vi "Get SMO Name.vi"(8 "error in (no error)":errorcluster, 11 "Example Instrument in":refnum<class "Instrument.Framework-Template.lvclass">) -> (0 "error out":errorcluster, 2 "SMO Name":string, 3 "Example Instrument out":refnum<class "Instrument.Framework-Template.lvclass">)   [LabVIEW 2019, in "Instrument.Framework-Template.lvclass"]
uses:
  Instrument.Framework-Template.lvclass
  Instrument Types/VSource/Instrument.VSource.lvclass
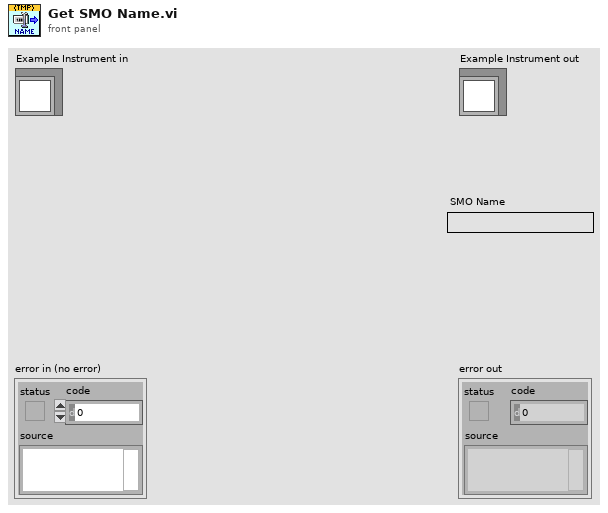
[diagram p1: front panel]
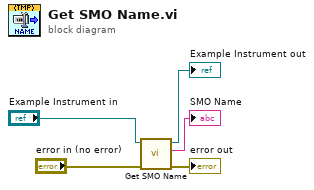
[diagram p0: block diagram]
diagram:
  n1 = call-parent "Get SMO Name.vi"("error in (no error)"="error in (no error)", "Instrument in"="Example Instrument in") -> ("error out"=→"error out":errorcluster, "SMO Name"=→"SMO Name":string, "Instrument out"=→"Example Instrument out":refnum<class "Instrument.Framework-Template.lvclass">)  [unwired: 7 in]
